vi "GetAlarms.vi"(0 "PM_Group in":refnum<class "PM_Group.lvclass">, 11 "error in (no error)":errorcluster) -> (4 "PM_Group out":refnum<class "PM_Group.lvclass">, 6 "Alarm":bool, 8 "Warning":bool, 15 "error out":errorcluster)   [LabVIEW 2019, in "PM_Group.lvclass"]
uses:
  PM_Group.lvclass
  PM_Group.lvclass/PM_Group.ctl
  Engine_1DO_2DI_class/Engine_1DO_2DI.lvclass
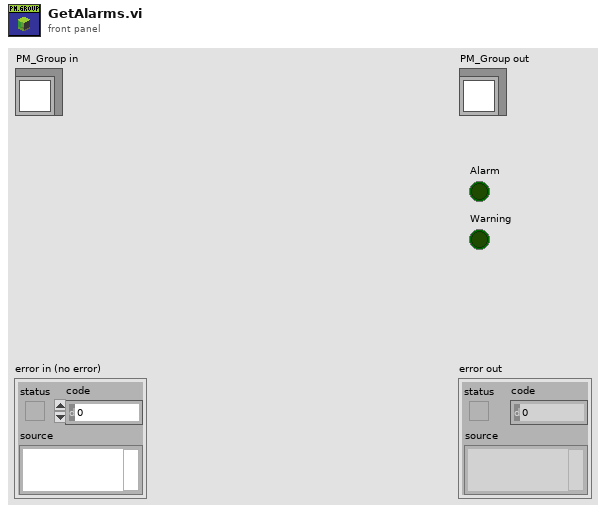
[diagram p1: front panel]
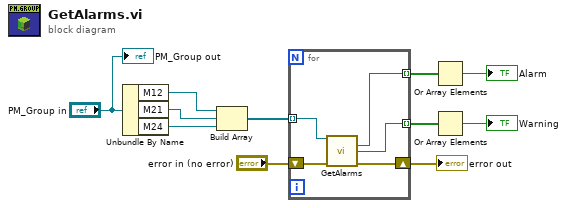
[diagram p0: block diagram]
diagram:
  n1 = Unbundle By Name("PM_Group in") -> ("M12"=w8:refnum<class "Engine_1DO_2DI.lvclass">, "M21"=w9:refnum<class "Engine_1DO_2DI.lvclass">, "M24"=w10:refnum<class "Engine_1DO_2DI.lvclass">)
  n2 = Build Array(w8, w9, w10) -> (w7:refnum<class "Engine_1DO_2DI.lvclass">[])
  n3 = for {
    tunnel: w7 -> [w16] mode=indexing
    shift-right: [w14] -> w5
    shift-left: "error in (no error)" -> [w15]
    tunnel: [w13] -> w4 mode=indexing
    tunnel: [w12] -> w3 mode=indexing
    n4 = call-dynamic "GetAlarms.vi"("Engine_1DO_2DI in"=w16, "error in (no error)"=w15) -> ("Alarm"=w13:bool, "Warning"=w12:bool, "error out"=w14:errorcluster)  [unwired: 10 in, 1 out]
  }
  "error out" <- w5
  n5 = Or Array Elements(Boolean array=w4) -> (logical OR=→"Alarm":bool)
  n6 = Or Array Elements(Boolean array=w3) -> (logical OR=→"Warning":bool)
  "PM_Group out" <- "PM_Group in"
